vi "ValveController.vi"(0 "Solenoid NC/NO":bool[](array[boolean]), 1 "Relay NO/NC":bool[](array[boolean])) -> ()   [LabVIEW 2021]
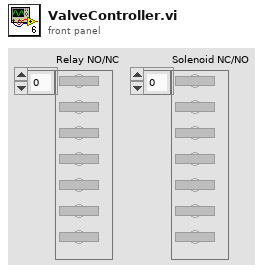
[diagram p1: front panel]
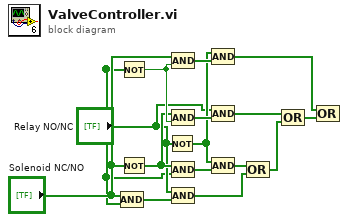
[diagram p0: block diagram]
diagram:
  n1 = Not(x="Solenoid NC/NO") -> (.not. x?=w6:bool[])
  n2 = Compound Arithmetic op=AND("Solenoid NC/NO") -> (w4:bool[], w2:bool[])
  n3 = Not(x=w2) -> (.not. x?=w14:bool)
  n4 = Not(x="Relay NO/NC") -> (.not. x?=w8:bool[])
  n5 = Compound Arithmetic op=AND("Solenoid NC/NO", w14) -> (w17:bool[])
  n6 = Compound Arithmetic op=AND(w6, w14) -> (w15:bool[])
  n7 = Compound Arithmetic op=AND(w6, w2) -> (w7:bool[])
  n8 = Compound Arithmetic op=AND("Relay NO/NC", w4) -> (w9:bool[])
  n9 = Compound Arithmetic op=AND(w8, w17) -> (w16:bool[])
  n10 = Compound Arithmetic op=AND("Relay NO/NC", w15) -> (w12:bool[])
  n11 = Compound Arithmetic op=AND(w8, w7) -> (w10:bool[])
  n12 = Compound Arithmetic op=OR(w10, w9) -> (w11:bool[])
  n13 = Compound Arithmetic op=OR(w12, w11) -> (w13:bool[])
  n14 = Compound Arithmetic op=OR(w16, w13) -> (w1:bool[])
